vi "ICM Buses Path.vi"() -> (0 "error out":errorcluster, 3 "ICM Buses Path":path)   [LabVIEW 2015]
doc: "ICM Buses Path.vi\n\nThis VI defines where the ICM Buses directory is located.\n\nInstrument Communication Module Version 1.0\nJuly, 2017 Original Code Consulting David Thomson\n www.originalcode.com"
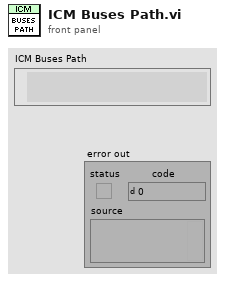
[diagram p1: front panel]
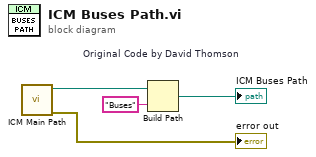
[diagram p0: block diagram]
diagram:
  w3 = "Buses"  # Original Code by David Thomson
  n1 = call "ICM Main Path.vi"() -> ("error out"=→"error out":errorcluster, "ICM Path"=w2:path)  [unwired: 10 in]
  n2 = Build Path(base path=w2, name or relative path=w3) -> (appended path=→"ICM Buses Path":path)
